vi "Durability_will_2012_07_10_main.vi"() -> ()   [LabVIEW 2011]
panel:
  out "error out":errorcluster
  in  "Speed 2/3":i8(slide)=100 min=0 max=100 step=10 scale=0.0..100.0
  in  "Speed 1":i8(slide)=50 min=0 max=100 step=10 scale=0.0..100.0
  in  "Motor 3":bool
  in  "Motor 2":bool
  in  "Motor 1":bool=TRUE
  in  "Quit 4":bool
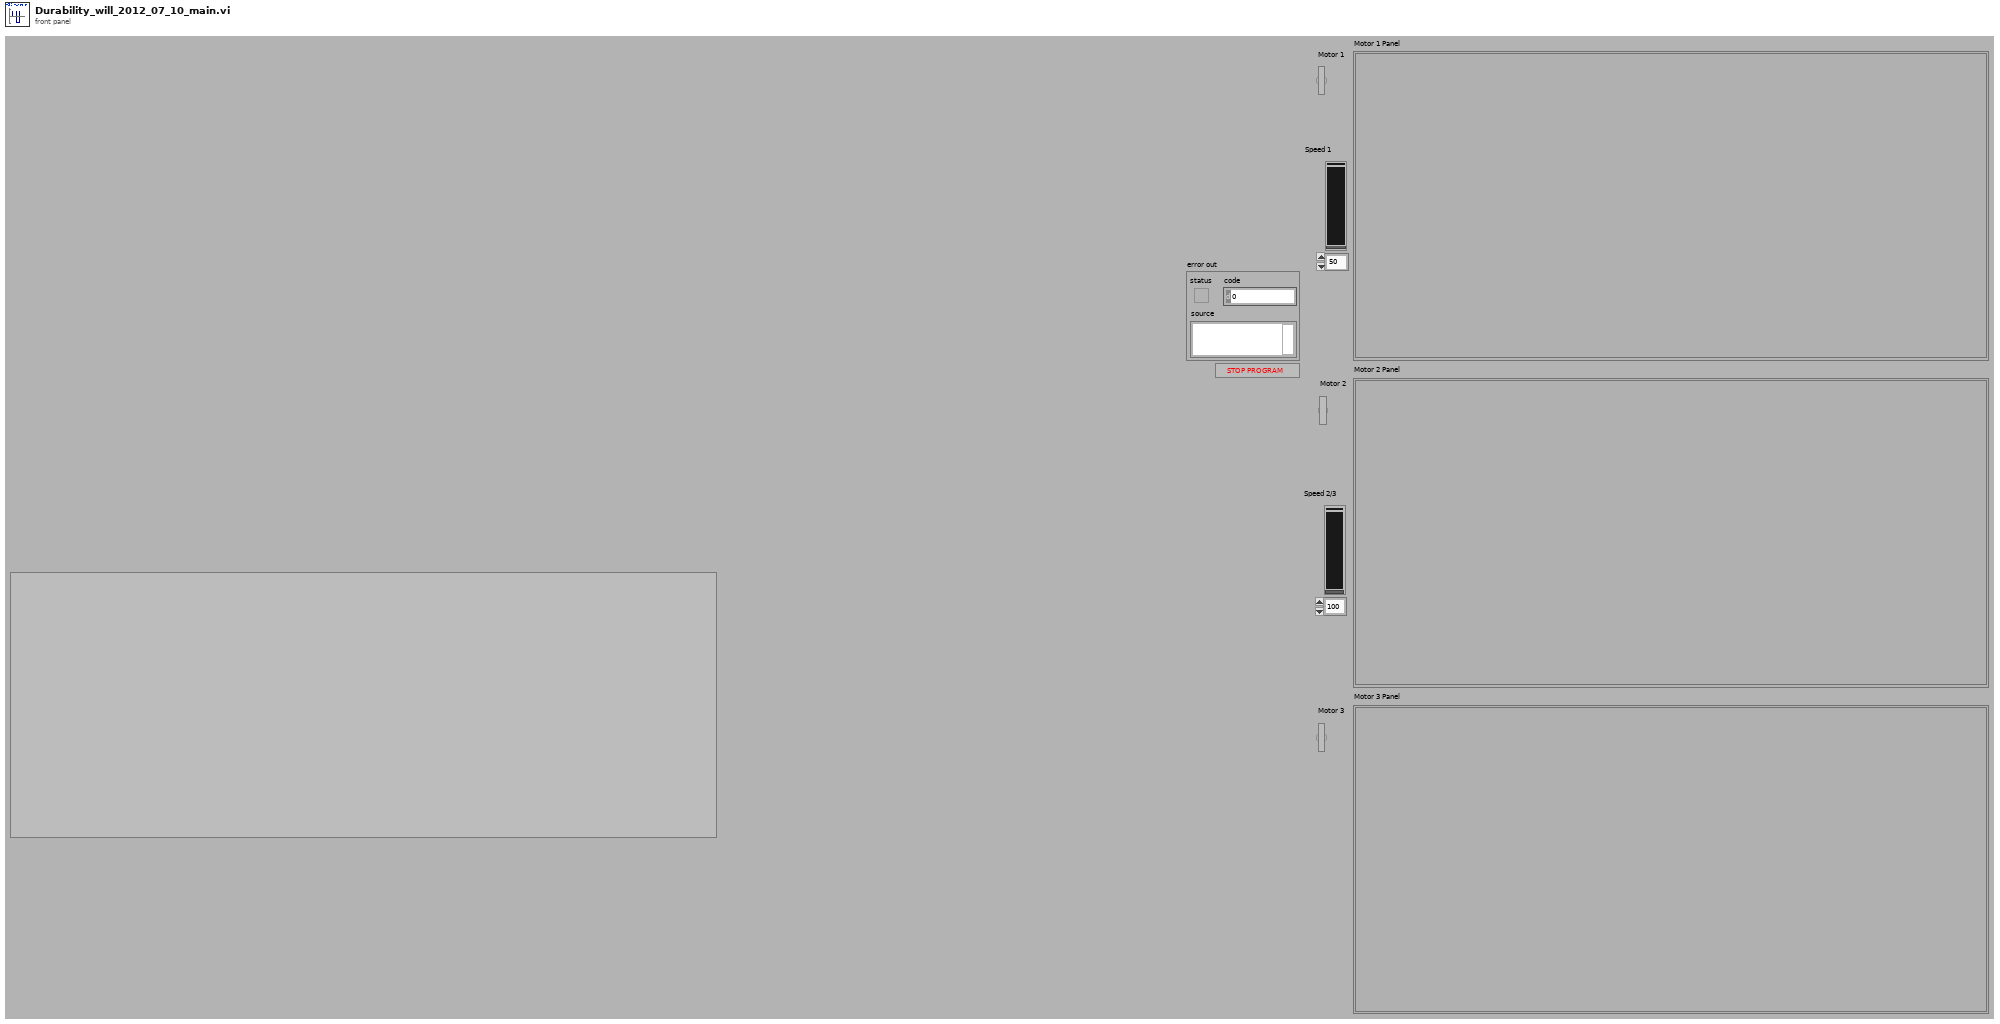
[diagram p1: front panel]
types:
  T1 = enum8{"Enabled", "Disabled", "Disabled and Grayed Out"}
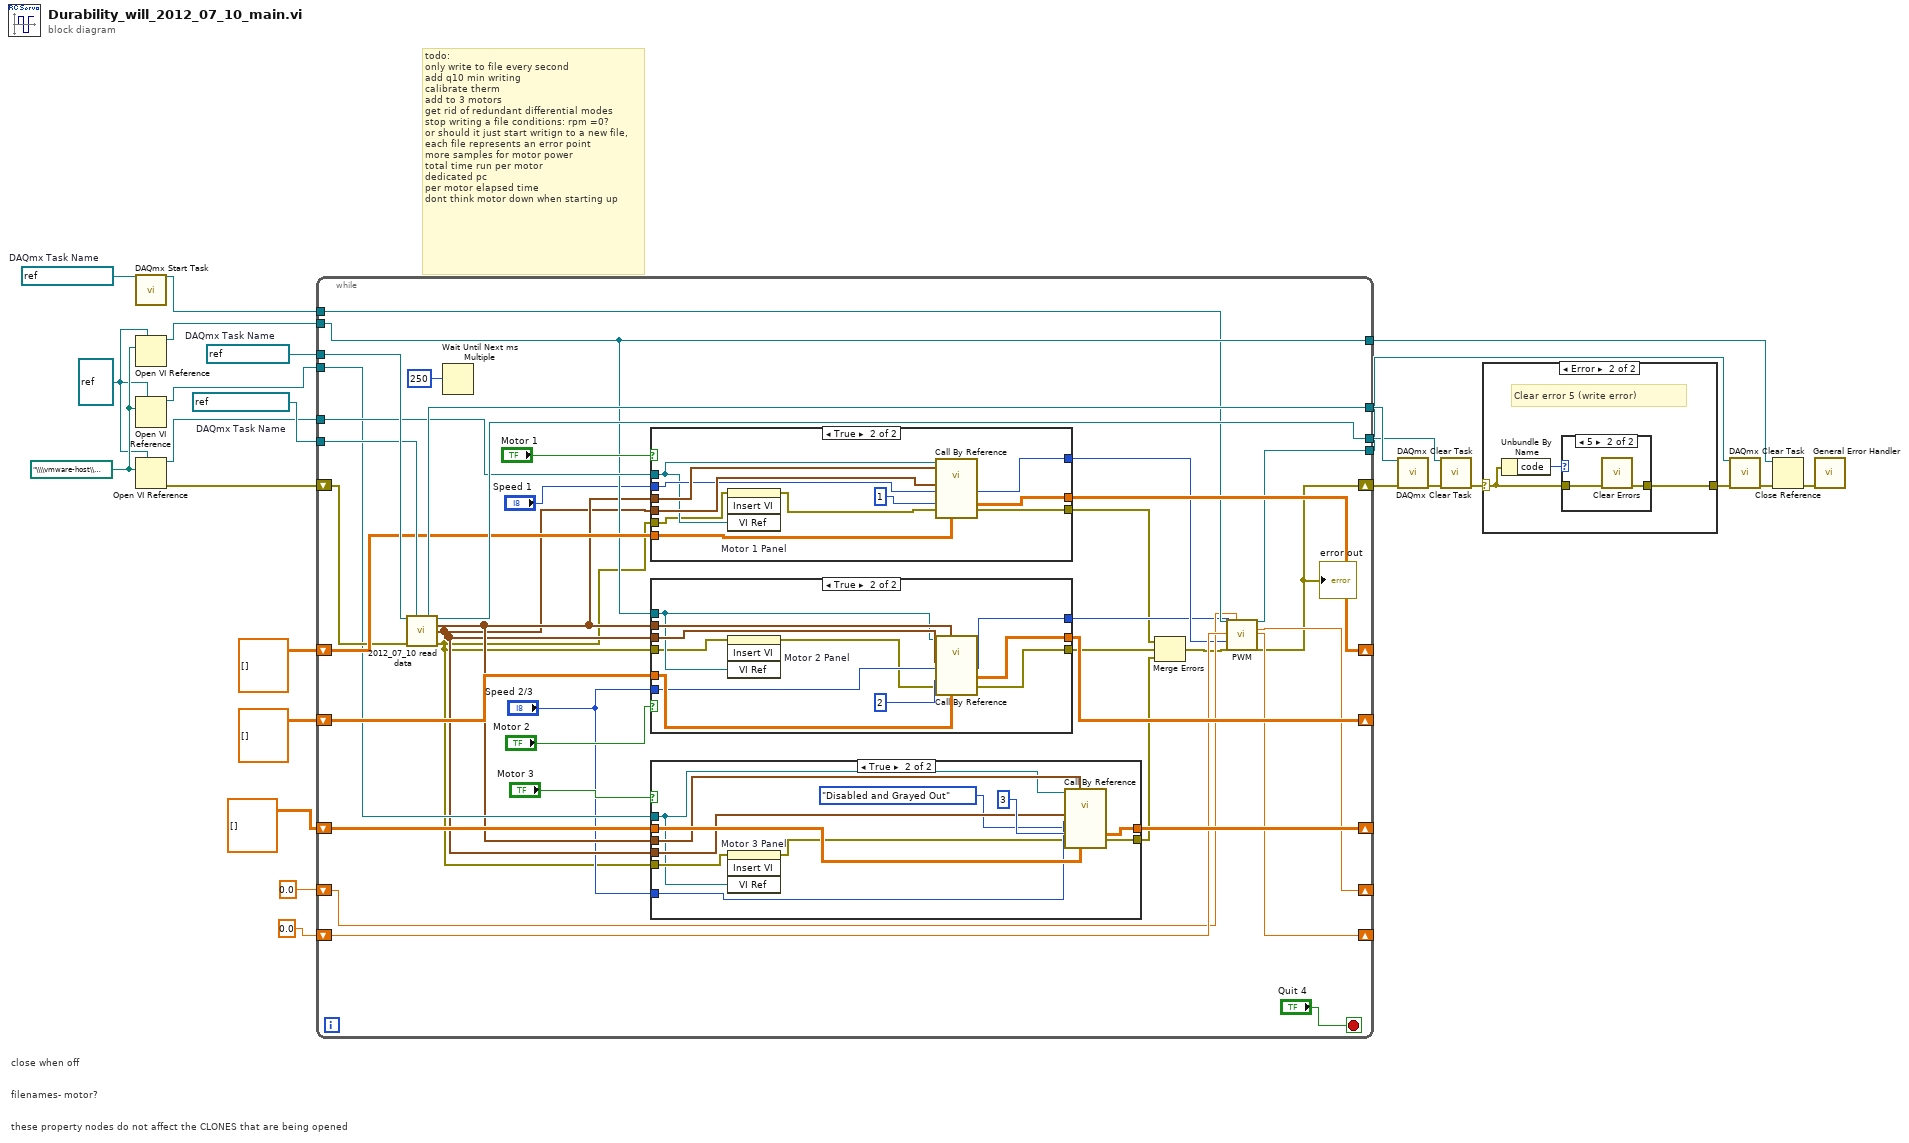
[diagram p0: block diagram]
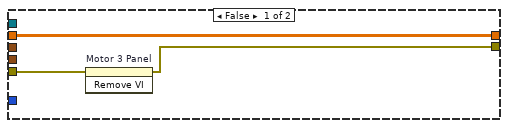
[diagram p4: hidden frame]
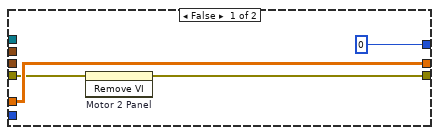
[diagram p5: hidden frame]
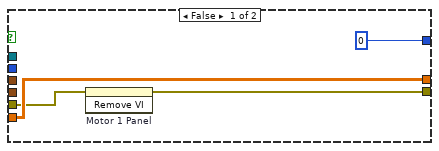
[diagram p6: hidden frame]
diagram:
  w6 = refnum<vi> refnum ("type specifier VI Refnum (for type only)")
  w7 = path "\\\\vmware-host\\Shared Folders/wclifton1/Google Drive/Procyrion/Durability/Durability Will/SubVIs/2012_07_10_each motor.vi" ("vi path")
  w10 = refnum<k21> "PWM Signal"  # DAQmx Task Name
  w24 = refnum<k21> "MC Power"  # DAQmx Task Name
  w25 = refnum<k21> "Motor Power"  # DAQmx Task Name
  # "filenames- motor?"
  # "close when off"
  # "these property nodes do not affect the CLONES that are being opened"
  # "todo:\nonly write to file every second\nadd q10 min writing\ncalibrate therm\nadd to 3 motors\nget rid of redundant differential modes\nstop writing a file conditions: rpm =0?\nor should it just start writign to a new file,\neach file represents an error point\nmore samples for motor power\ntotal time run per motor\ndedicated pc\nper motor elapsed time\ndont think motor down when starting up"
  n1 = call <vilib>:"DAQmx Start Task.vi"("task/channels in"=w10) -> ("task out"=w8:refnum<k21>)  [unwired: 13 in, 1 out]
  n2 = Open VI Reference(type specifier VI Refnum (for type only)=w6, vi path=w7) -> (vi reference=w2:refnum<vi>)  [unwired: 4 in, 1 out]
  n3 = Open VI Reference(type specifier VI Refnum (for type only)=w6, vi path=w7) -> (vi reference=w1:refnum<vi>)  [unwired: 4 in, 1 out]
  n4 = Open VI Reference(type specifier VI Refnum (for type only)=w6, vi path=w7) -> (vi reference=w3:refnum<vi>, error out=w9:errorcluster)  [unwired: 4 in]
  n5 = while {
    tunnel: w24 -> [w60]
    tunnel: w25 -> [w59]
    shift-right: [w55] -> _
    shift-left: dbl[][][] [] -> [w56]
    shift-right: [w28] -> w23
    shift-left: w9 -> [w48]
    shift-right: [w35] -> _
    shift-left: 0.0 -> [w36]
    tunnel: [w58] -> w17
    tunnel: [w57] -> w16
    shift-right: [w52] -> _
    shift-left: dbl[][][] [] -> [w53]
    shift-right: [w34] -> _
    shift-left: 0.0 -> [w37]
    tunnel: w3 -> [w51]
    tunnel: [w49] -> w13
    tunnel: w2 -> [w49]
    tunnel: w8 -> [w47]
    shift-right: [w46] -> _
    shift-left: dbl[][][] [] -> [w45]
    tunnel: w1 -> [w44]
    tunnel: [w40] -> w5
    stop <- "Quit 4" stop-if-true
    n6 = call "2012_07_10 read data.vi"("MC Power"=w60, "Motor Power"=w59, "Error In"=w48) -> ("Motor Power Out"=w58:refnum<k21>, "MC Power Out"=w57:refnum<k21>, "Motor Power Data"=w42:waveform(dbl)[], "MC Power Data"=w41:waveform(dbl)[], "error out"=w31:errorcluster)  [unwired: 8 in]
    n7 = Wait Until Next ms Multiple(millisecond multiple=u32 250) -> ()  [unwired: 1 out]
    n8 = case shown="True" "Motor 1" {
      tunnel: [w93 w101] -> w26
      tunnel: w31 -> [w92 w97]
      tunnel: w56 -> [w95 w105]
      tunnel: [w95 w106] -> w55
      tunnel: w41 -> [_ w103]
      tunnel: w42 -> [_ w102]
      tunnel: w51 -> [_ w98]
      tunnel: "Speed 1" -> [_ w100]
      tunnel: [i8 0 ("Power \nSetting") w99] -> w33
      frame False {
        n9 = invoke on="Motor 1 Panel" class="SubPnl" method="Remove VI"(error in=w92) -> (error out=w93:errorcluster)  [unwired: 2 in, 2 out]
      }
      frame True {
        n10 = invoke on="Motor 1 Panel" class="SubPnl" method="Insert VI"(error in=w97, "VI Ref"=w98) -> (error out=w96:errorcluster)  [unwired: 2 in, 3 out]
        n11 = call-by-ref "?"(reference=w98, "MC Power Data In"=w103, "Motor Power Data In"=w102, "Power \nSetting"=w100, "Motor"=i16 1, "Error In"=w96, "Fine Data In"=w105) -> ("Power \nSetting"=w99:i8, "Fine Data Out"=w106:dbl[][][], "Errors"=w101:errorcluster)  [unwired: 8 in, 2 out]
      }
    }
    n12 = case shown="True" "Motor 2" {
      tunnel: [w78 w91] -> w27
      tunnel: w53 -> [w80 w89]
      tunnel: [w80 w90] -> w52
      tunnel: w49 -> [_ w83]
      tunnel: w41 -> [_ w87]
      tunnel: w42 -> [_ w86]
      tunnel: w31 -> [w77 w82]
      tunnel: "Speed 2/3" -> [_ w85]
      tunnel: [i8 0 ("Power \nSetting") w84] -> w32
      frame False {
        n13 = invoke on="Motor 2 Panel" class="SubPnl" method="Remove VI"(error in=w77) -> (error out=w78:errorcluster)  [unwired: 2 in, 2 out]
      }
      frame True {
        n14 = invoke on="Motor 2 Panel" class="SubPnl" method="Insert VI"(error in=w82, "VI Ref"=w83) -> (error out=w81:errorcluster)  [unwired: 2 in, 3 out]
        n15 = call-by-ref "?"(reference=w83, "MC Power Data In"=w87, "Motor Power Data In"=w86, "Power \nSetting"=w85, "Motor"=i16 2, "Error In"=w81, "Fine Data In"=w89) -> ("Power \nSetting"=w84:i8, "Fine Data Out"=w90:dbl[][][], "Errors"=w91:errorcluster)  [unwired: 8 in, 2 out]
      }
    }
    n16 = case shown="True" "Motor 3" {
      tunnel: [w63 w76] -> w30
      tunnel: w45 -> [w65 w74]
      tunnel: [w65 w75] -> w46
      tunnel: w44 -> [_ w66]
      tunnel: w41 -> [_ w72]
      tunnel: w42 -> [_ w71]
      tunnel: w31 -> [w64 w68]
      tunnel: "Speed 2/3" -> [_ w70]
      frame False {
        n17 = invoke on="Motor 3 Panel" class="SubPnl" method="Remove VI"(error in=w64) -> (error out=w63:errorcluster)  [unwired: 2 in, 2 out]
      }
      frame True {
        n18 = invoke on="Motor 3 Panel" class="SubPnl" method="Insert VI"(error in=w68, "VI Ref"=w66) -> (error out=w67:errorcluster)  [unwired: 2 in, 3 out]
        n19 = call-by-ref "?"(reference=w66, "MC Power Data In"=w72, "Motor Power Data In"=w71, "Power \nSetting"=w70, "On/Off Control"=T1."Disabled and Grayed Out", "Motor"=i16 3, "Error In"=w67, "Fine Data In"=w74) -> ("Fine Data Out"=w75:dbl[][][], "Errors"=w76:errorcluster)  [unwired: 7 in, 3 out]
      }
    }
    n20 = Merge Errors(w26, w27, w30) -> (w29:errorcluster)
    n21 = call "PWM.vi"("Refnum in"=w47, "High Time In 2"=w37, "Speed 1"=w33, "Speed 2/3"=w32, "error in (no error)"=w29, "High Time In 1"=w36) -> ("Refnum out"=w40:refnum<k21>, "High Time Out 1"=w35:dbl, "High Time Out 2"=w34:dbl, "error out"=w28:errorcluster)  [unwired: 18 in]
    "error out" <- w28
  }
  n22 = call <vilib>:"DAQmx Clear Task.vi"("task in"=w17, "error in"=w23) -> ("error out"=w19:errorcluster)  [unwired: 13 in]
  n23 = call <vilib>:"DAQmx Clear Task.vi"("task in"=w16, "error in"=w19) -> ("error out"=w21:errorcluster)  [unwired: 13 in]
  n24 = case shown="Error" w21 {
    selector: w21 -> [w107 w109]
    tunnel: [w107 w108] -> w20
    frame No Error {
    }
    frame Error {
      # "Clear error 5 (write error)"
      n25 = Unbundle By Name(w109) -> ("code"=w110:i32)
      n26 = case shown="5" w110 {
        tunnel: w109 -> [w111 w113]
        tunnel: [w111 w112] -> w108
        frame Default {
        }
        frame 5 {
          n27 = call <vilib>:"Clear Errors.vi"("error in (no error)"=w113) -> ("error out"=w112:errorcluster)  [unwired: 6 in]
        }
      }
    }
  }
  n28 = call <vilib>:"DAQmx Clear Task.vi"("task in"=w5, "error in"=w20) -> ("error out"=w12:errorcluster)  [unwired: 13 in]
  n29 = Close Reference(reference=w13, error in (no error)=w12) -> (error out=w11:errorcluster)
  n30 = call <vilib>:"General Error Handler.vi"("error in (no error)"=w11) -> ()  [unwired: 10 in, 5 out]
